vi "HS_DAQ_FPGA.vi"() -> ()   [LabVIEW 2020]
uses:
  <vilib>/Platform/TimedLoop/XDataNode/timing_clust.ctl
  <vilib>/Platform/TimedLoop/XDataNode/nitl_modes.ctl
  <vilib>/Platform/TimedLoop/XDataNode/wakeup.ctl
  <vilib>/rvi/Emulation/niFpgaGetClockAttributes.vi
  <vilib>/rvi/Emulation/niFpgaSctlEmulationGetInTimedLoop.vi
  <vilib>/rvi/Emulation/niFpgaEmulationReportErrorSimple.vi
  <vilib>/rvi/eio/common/nirviEmuTemplateMethod_errors.vi
  <vilib>/rvi/interface/RandomDataEmulation/nirviRandomDataMultiElementFPGAFIFO.vi
  <instcachedir>/0/nirviRandomDataMultiElementFPGAFIFO_3E9965BA1FAD4E7B8DABA31768A09B1F.lvgen/nirviRandomDataMultiElementFPGAFIFO_3E9965BA1FAD4E7B8DABA31768A09B1F_003.vi
  <vilib>/rvi/interface/RandomDataEmulation/niFpgaRandomDataHandleErrors.vi
  <vilib>/rvi/Emulation/niFpgaEmulationIsFPGAContextNoSignature.vi
  <vilib>/rvi/DataTransferAndStorage/Container/Common/niFpgaContainerGetUniqueNameForEmu.vi
  <vilib>/rvi/Memory/Memory_Emulation/niFpgaMemoryEmulationCacheClearOnFirstRun.vi
  <vilib>/rvi/Memory/Memory_Emulation/nirvimemoryEmulationManagerCache_MakeExclusive.vi
  <vilib>/rvi/Memory/Memory_Emulation/niFpgaMemoryEmulationValidateCache.vi
  <vilib>/rvi/Memory/Memory_Emulation/nirvimemoryEmulationManagerCache_InsertValue.vi
  <vilib>/Utility/error.llb/Clear Errors.vi
  <vilib>/rvi/Memory/Memory_Emulation/nirvimemoryEmulationManagerCache_ReleaseExclusive.vi
  <vilib>/rvi/Memory/Memory_Emulation/nirvimemoryEmulationManagerCache_GetValue.vi
  <vilib>/rvi/Memory/Memory_Emulation/nirvimemoryEmulationManagerCache_SetValue.vi
  <vilib>/rvi/Emulation/niFpgaProcessEmulError.vi
  <vilib>/rvi/Emulation/niFpgaCriticalErrorInLSC.vi
  <vilib>/eio/EIONode/EIONode.xnode
  <vilib>/rvi/DataTransferAndStorage/Container/XNode/niFpgaContainer.xnode
  <vilib>/rvi/interface/RandomDataEmulation/nirviRandomDataFpgaMultiElementTemplate.vi
  <vilib>/rvi/DataTransferAndStorage/Register/Emulation/niFpgaRegisterEmulation.vi
  <vilib>/rvi/interface/RandomDataEmulation/nirviRandomDataFpgaReadWriteTemplate.vi
  <vilib>/platform/TimedLoop/XDataNode/XDataNode.xnode
  <vilib>/Platform/TimedLoop/XDataNode/XDNodeRunTimeDep.lvlib
panel:
  out "Mod3/CJC0":fxp<+/-,24,-2>
  out "Mod3/Autozero":fxp<+/-,24,-2>
  out "TC0":fxp<+/-,24,-2>
  out "FPGA temp loop time [ticks]":u32
  in  "Temp sample period [ticks]":u32=40000000
  out "DigitalData":u32[](array[numeric])
  out "FPGA analog loop time [ticks]":u32
  out "AnalogData":fxp<+/-,26,5>[](array[numeric])
  out "PulseCount":u32
  out "Period":u32
  in  "Analog sample period [ticks]":u32=4000
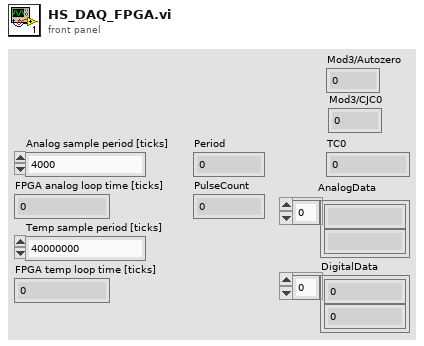
[diagram p1: front panel]
types:
  T1 = typedef "XDNodeRunTimeDep.lvlib/timing_clust.ctl" = cluster{"Expected End [f-1]":u64, "Actual End [f-1]":u64, "Finished Late? [f-1]":bool, "Expected End [i-1]":u64, "Actual End [i-1]":u64, "Finished Late? [i-1]":bool, "Expected Start [i]":u64, "Actual Start [i]":u64, "Expected Start [f]":u64, "Actual Start [f]":u64, "Source Name":string, "Structure Name":string, "Period":i64, "Deadline":i64, "Offset":i64, "Start":i64, "Priority":i32, "Timeout":i32, "Mode":T2, "Wakeup Reason":T3, "Error":errorcluster, "Source Type":string, "Secondary Source Type":string, "Global End Time":u64, "Global Start Time":u64, "Frame Duration":u64, "Iteration Duration":u64, "Assigned CPU":i32, "I/O Scan Engine Mode":u32}
  T2 = typedef "XDNodeRunTimeDep.lvlib/nitl_modes.ctl" = enum32{"No Change", "Process missed periods, maintain original phase", "Discard missed periods, maintain original phase", "Process missed periods, ignore original phase", "Discard missed periods, ignore original phase"}
  T3 = typedef "XDNodeRunTimeDep.lvlib/wakeup.ctl" = enum32{"Normal", "Aborted", "Asynchronous wakeup", "Timing source error", "Timed loop error", "Timeout"}
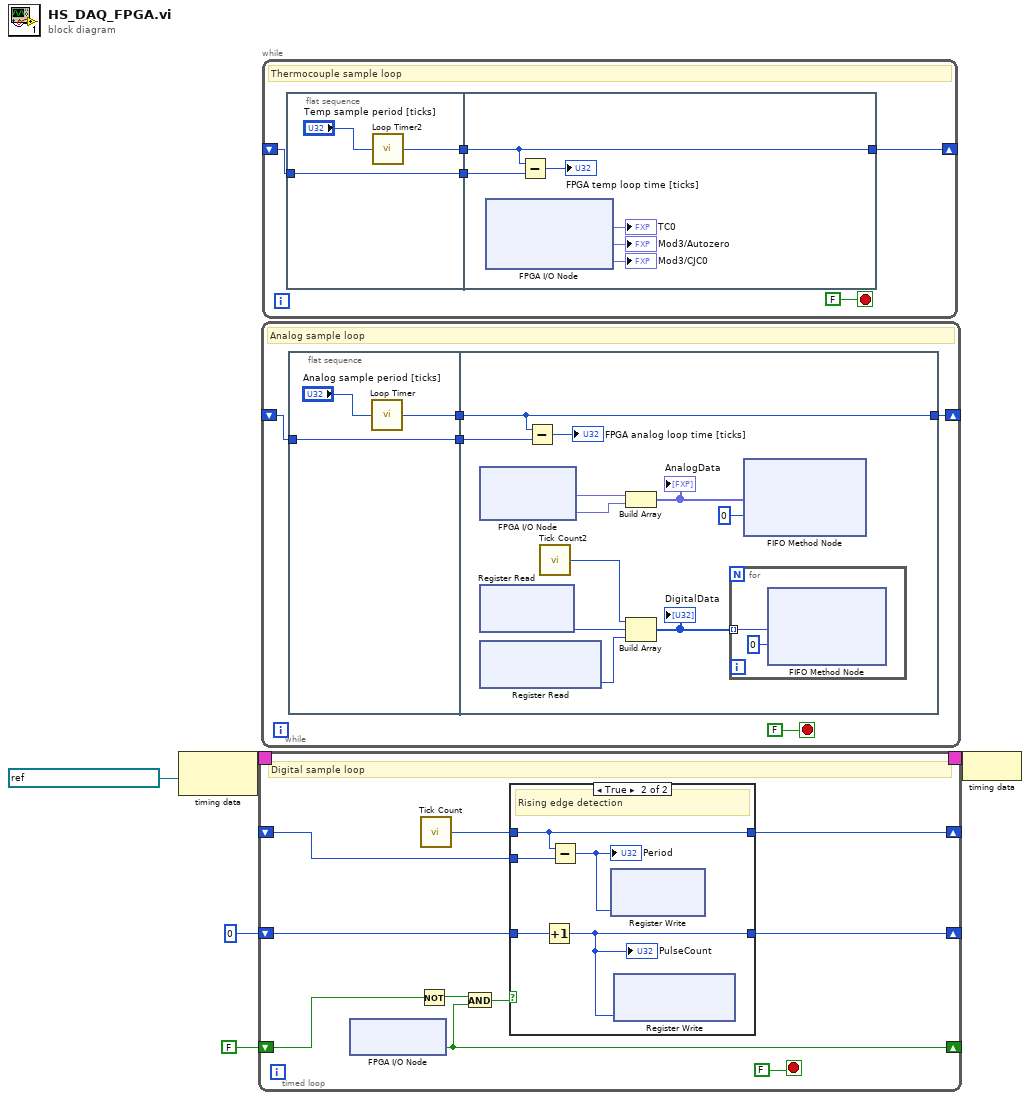
[diagram p0: block diagram]
diagram:
  n1 = node-c288(refnum<k21> "40 MHz Onboard Clock" ("Source Name")) -> (w5:T1)
  n2 = timed-loop {
    timing: w5 -> [_]
    timing-out: [_] -> w4
    shift-right: [w14] -> _
    shift-left: FALSE ("Mod2/DI0") -> [w13]
    shift-right: [w10] -> _
    shift-left: _ -> [w9]
    shift-right: [w6] -> _
    shift-left: u32 0 -> [w7]
    stop <- FALSE stop-if-true
    # "Digital sample loop"
    n3 = xnode "FPGA I/O Node"() -> ("Mod2/DI0"=w14:bool)  [unwired: 1 in, 1 out]
    n4 = Not(x=w13) -> (.not. x?=w15:bool)
    n5 = call "Tick Count"() -> ("Tick Count(Ticks)"=w11:u32)
    n6 = And(x=w15, y=w14) -> (x .and. y?=w12:bool)
    n7 = case shown="True" w12 {
      tunnel: w11 -> [_ w22]
      tunnel: [w17 w22] -> w10
      tunnel: w9 -> [w17 w21]
      tunnel: w7 -> [w16 w19]
      tunnel: [w16 w18] -> w6
      frame False {
      }
      frame True {
        # "Rising edge detection"
        n8 = Increment(x=w19) -> (x+1=w18:u32)
        "PulseCount" <- w18
        n9 = Subtract(x=w22, y=w21) -> (x-y=w20:u32)
        "Period" <- w20
        n10 = xnode ("Register Write")("Data"=w20) -> ()  [unwired: 1 in, 1 out]
        n11 = xnode ("Register Write")("Data"=w18) -> ()  [unwired: 1 in, 1 out]
      }
    }
  }
  n12 = while {
    shift-right: [w27] -> _
    shift-left: _ -> [w26]
    stop <- FALSE stop-if-true
    # "Analog sample loop"
    n13 = flat-sequence {
      tunnel: [w31] -> w28
      tunnel: w26 -> [w30]
      tunnel: [w30] -> w25
      tunnel: w28 -> [w37]
      tunnel: [w37] -> w27
      tunnel: w25 -> [w36]
      frame #0 {
        n14 = call "Loop Timer"("Count(Ticks)"="Analog sample period [ticks]") -> ("Tick Count(Ticks)"=w31:u32)
      }
      frame #1 {
        n15 = xnode "FPGA I/O Node"() -> ("Mod1/AI0"=w43:fxp<+/-,26,5>, "Mod1/AI1"=w42:fxp<+/-,26,5>)  [unwired: 2 in, 2 out]
        n16 = xnode ("Register Read")() -> ("Data"=w39:u32)  [unwired: 1 in, 1 out]
        n17 = xnode ("Register Read")() -> ("Data"=w38:u32)  [unwired: 1 in, 1 out]
        n18 = Subtract(x=w37, y=w36) -> (x-y=→"FPGA analog loop time [ticks]":u32)
        n19 = call "Tick Count2"() -> ("Tick Count(uSec)"=w34:u32)
        n20 = Build Array(w43, w42) -> (w41:fxp<+/-,26,5>[])
        "AnalogData" <- w41
        n21 = Build Array(w34, w39, w38) -> (w33:u32[])
        "DigitalData" <- w33
        n22 = for {
          tunnel: w33 -> [w44] mode=indexing
          n23 = xnode ("FIFO Method Node")("Element"=w44, "Timeout"=0) -> ()  [unwired: 1 in, 2 out]
        }
        n24 = xnode ("FIFO Method Node")("Element"=w41, "Timeout"=0) -> ()  [unwired: 1 in, 2 out]
      }
    }
  }
  n25 = while {
    shift-right: [w48] -> _
    shift-left: _ -> [w47]
    stop <- FALSE stop-if-true
    # "Thermocouple sample loop"
    n26 = flat-sequence {
      tunnel: [w52] -> w49
      tunnel: w47 -> [w51]
      tunnel: [w51] -> w46
      tunnel: w49 -> [w59]
      tunnel: [w59] -> w48
      tunnel: w46 -> [w58]
      frame #0 {
        n27 = call "Loop Timer2"("Count(Ticks)"="Temp sample period [ticks]") -> ("Tick Count(Ticks)"=w52:u32)
      }
      frame #1 {
        n28 = xnode "FPGA I/O Node"() -> ("Mod3/TC0"=→"TC0":fxp<+/-,24,-2>, "Mod3/Autozero"=→"Mod3/Autozero":fxp<+/-,24,-2>, "Mod3/CJC0"=→"Mod3/CJC0":fxp<+/-,24,-2>)  [unwired: 3 in, 3 out]
        n29 = Subtract(x=w59, y=w58) -> (x-y=→"FPGA temp loop time [ticks]":u32)
      }
    }
  }
  n30 = node-c288(w4) -> ()
